vi "Get All Devices.vi"(8 "error in (no error)":errorcluster, 11 "HAL Manager in":refnum<class "HAL Manager.lvclass">) -> (0 "error out":errorcluster, 2 "Devices":refnum<class "Device.lvclass">[](array[class]), 3 "HAL Manager out":refnum<class "HAL Manager.lvclass">)   [LabVIEW 2012, in "HAL.lvlib" / "HAL Manager.lvclass"]
uses:
  HAL Manager.lvclass
  Device/Device.lvclass
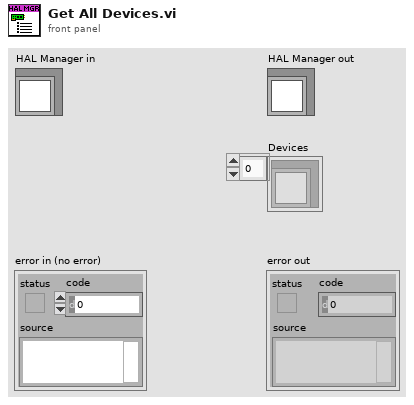
[diagram p1: front panel]
types:
  T1 = typedef "HAL.lvlib/HAL Manager.lvclass/Ref Data.ctl" = cluster{"Devices":refnum<class "Device.lvclass">[], "Type":string[], "Models":string[], "Name":string[]}
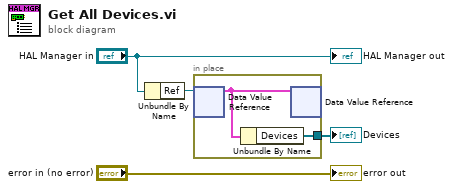
[diagram p0: block diagram]
diagram:
  n1 = Unbundle By Name("HAL Manager in") -> ("Ref"=w3:refnum<data-value>)
  n2 = in-place {
    in-place-border: [w5] -> w1
    n3 = in-place-dvr #1(w3) -> (w6:T1)  [unwired: 1 out]
    n4 = Unbundle By Name(w6) -> ("Devices"=w5:refnum<class "Device.lvclass">[])
    n5 = in-place-dvr #1(w6) -> ()  [unwired: 2 out]
  }
  "Devices" <- w1
  "error out" <- "error in (no error)"
  "HAL Manager out" <- "HAL Manager in"
